vi "Configure Measurement (Power Meter - Zeroing).vi"(0 "VISA resource name":refnum<visa-resource-name>, 5 "Zeroing Type (0: External)":i32(ring) items=["External", "Internal"], 11 "error in (no error)":errorcluster) -> (4 "VISA resource name out":refnum<visa-resource-name>, 15 "error out":errorcluster)   [LabVIEW 2022 SP3, in "Agilent N934X Series.lvlib"]
doc: "Configures the cable setting of Power Meter Zeroing.\n\nNotes:\n(1) Option PWM or PWP is required to enable this function. Option PWM supports Keysight (Agilent) U2000 series USB average power sensor, and Option PWP supports Keysight (Agilent) U2020 X series peak power sensor.\n\n(2) This VI is only applicable for N9321C, N9322C, N9323C, N9324C models"
uses:
  <instrlib>/Agilent N934X Series/Agilent N934X Series.lvlib
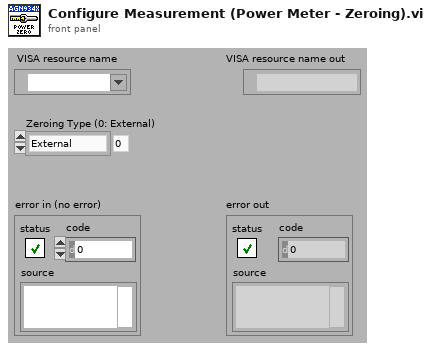
[diagram p1: front panel]
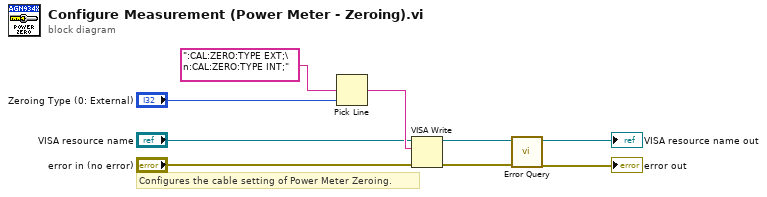
[diagram p0: block diagram]
diagram:
  # "Configures the cable setting of Power Meter Zeroing."
  n1 = Pick Line(multi-line string=":CAL:ZERO:TYPE EXT;\n:CAL:ZERO:TYPE INT;", line index="Zeroing Type (0: External)") -> (output string=w7:string)  [unwired: 1 in]
  n2 = VISA Write(VISA resource name="VISA resource name", write buffer=w7, error in (no error)="error in (no error)") -> (VISA resource name out=w4:refnum<visa-resource-name>, error out=w3:errorcluster)  [unwired: 1 out]
  n3 = call <instrlib>:"Error Query.vi"("error in (no error)"=w3, "VISA resource name"=w4) -> ("error out"=→"error out":errorcluster, "VISA resource name out"=→"VISA resource name out":refnum<visa-resource-name>)  [unwired: 6 in, 2 out]
